vi "Acquire Image.vi"(8 "error in (no error)":errorcluster, 9 "Cluster":T1={"Bayer"={"Algorithm"=0, "Gain R"=1.0, "Gain B"=1.0, "Gain G"=1.0, "Pattern"=5}, "Acquisition Control"={"Trigger Selector"=0, "Acquisition Frame Rate"=0.0, "Exposure Time"=0.0, "Acquisition Frame Rate Target"=0.0}, "Analog Control"={"Black Level"=1.5, "Gain Selector"=10, "Gain"=1.0}} {"Analog Control"."Gain" min=1.0 max=15.0; "Analog Control"."Gain Selector" items=["Analog All"=10, "Digital All"=20]; "Analog Control"."Black Level" min=0.0 max=255.9375; "Acquisition Control"."Acquisition Frame Rate Target" min=0.001 max=150000000.0; "Acquisition Control"."Exposure Time" min=27.793333333333333 max=1048539.7933333333; "Acquisition Control"."Acquisition Frame Rate" min=0.9536888685435264 max=30.757874015748033; "Acquisition Control"."Trigger Selector" items=["Frame Start"=3, "Exposure Start"=10]; "Bayer"."Pattern" items=["Use hardware value"=5, "None"=0, "GB"=1, "GR"=2, "BG"=3, "RG"=4]; "Bayer"."Gain G" min=0.0 max=3.999; "Bayer"."Gain B" min=0.0 max=3.999; "Bayer"."Gain R" min=0.0 max=3.999; "Bayer"."Algorithm" items=["Bilinear", "VNG"]}, 10 "Stop":bool, 11 "Edmund Optics in":refnum<class "Edmund Optics.lvclass">) -> (0 "error out":errorcluster, 2 "Image Out":T2(plugin-control), 3 "Edmund Optics out":refnum<class "Edmund Optics.lvclass">)   [LabVIEW 2021, in "Edmund Optics.lvclass"]
uses:
  Edmund Optics.lvclass
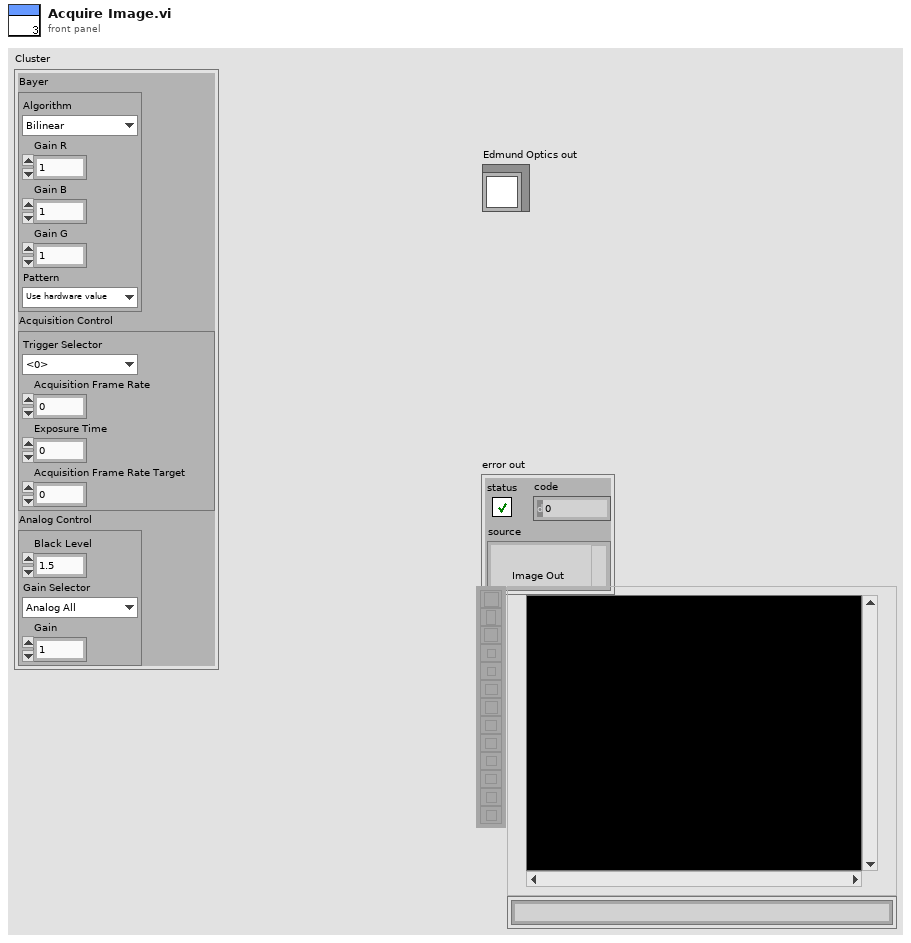
[diagram p1: front panel]
types:
  T1 = cluster{"Bayer":cluster{"Algorithm":u32, "Gain R":dbl, "Gain B":dbl, "Gain G":dbl, "Pattern":u32}, "Acquisition Control":cluster{"Trigger Selector":u32, "Acquisition Frame Rate":dbl, "Exposure Time":dbl, "Acquisition Frame Rate Target":dbl}, "Analog Control":cluster{"Black Level":dbl, "Gain Selector":u32, "Gain":dbl}}
  T2 = typedef "IMAQ Image.ctl" = refnum<image>
  T3 = cluster{"Algorithm":u32, "Gain R":dbl, "Gain B":dbl, "Gain G":dbl, "Pattern":u32}
  T4 = cluster{"Trigger Selector":u32, "Acquisition Frame Rate":dbl, "Exposure Time":dbl, "Acquisition Frame Rate Target":dbl}
  T5 = cluster{"Black Level":dbl, "Gain Selector":u32, "Gain":dbl}
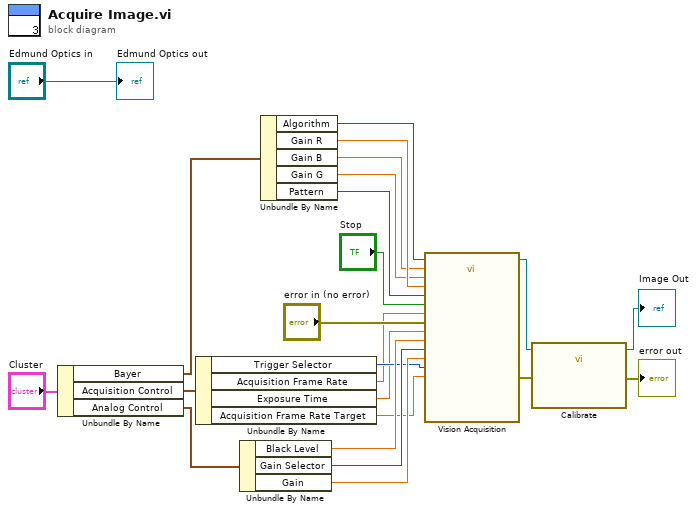
[diagram p0: block diagram]
diagram:
  n1 = Unbundle By Name("Cluster") -> ("Bayer"=w15:T3, "Acquisition Control"=w14:T4, "Analog Control"=w13:T5)
  n2 = Unbundle By Name(w14) -> ("Trigger Selector"=w4:u32, "Acquisition Frame Rate"=w3:dbl, "Exposure Time"=w2:dbl, "Acquisition Frame Rate Target"=w1:dbl)
  n3 = Unbundle By Name(w13) -> ("Black Level"=w7:dbl, "Gain Selector"=w6:u32, "Gain"=w5:dbl)
  n4 = Unbundle By Name(w15) -> ("Algorithm"=w12:u32, "Gain R"=w11:dbl, "Gain B"=w10:dbl, "Gain G"=w9:dbl, "Pattern"=w8:u32)
  n5 = call "Vision Acquisition"("Bayer::Algorithm"=w12, "Bayer::Gain B"=w10, "Bayer::Gain G"=w9, "Bayer::Gain R"=w11, "Bayer::Pattern"=w8, "Stop (F)"="Stop", "Acquisition Control::Acquisition Frame Rate"=w3, "error in"="error in (no error)", "Acquisition Control::Acquisition Frame Rate Target"=w1, "Acquisition Control::Exposure Time"=w2, "Acquisition Control::Trigger Selector"=w4, "Analog Control::Black Level"=w7, "Analog Control::Gain"=w5, "Analog Control::Gain Selector"=w6) -> ("Image Out"=w23:T2, "error out"=w22:errorcluster)  [unwired: 11 in, 1 out]
  n6 = call "Calibrate"("Image In"=w23, "error in"=w22) -> ("Image Out"=→"Image Out":T2, "error out"=→"error out":errorcluster)  [unwired: 24 in]
  "Edmund Optics out" <- "Edmund Optics in"
